vi "ABB Roundoff.vi"(10 "Precision":i32, 11 "# in":dbl) -> (3 "# out":dbl)   [LabVIEW 2017]
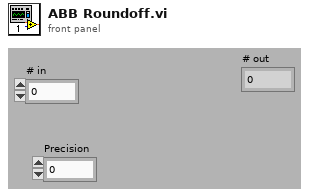
[diagram p1: front panel]
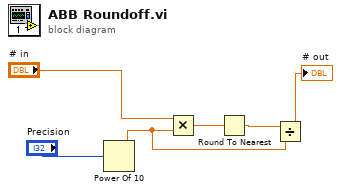
[diagram p0: block diagram]
diagram:
  n1 = Power Of 10(x="Precision") -> (10^x=w2:dbl)
  n2 = Multiply(x="# in", y=w2) -> (x*y=w4:dbl)
  n3 = Round To Nearest(number=w4) -> (nearest integer value=w3:dbl)
  n4 = Divide(x=w3, y=w2) -> (x/y=→"# out":dbl)
